vi "Change Bookmarks Type.vi"(8 "Error In":errorcluster, 10 "Data":variant, 11 "State In":T1) -> (0 "Error Out":errorcluster, 3 "State Out":T1)   [LabVIEW 2017, in "Graveyard.lvlib"]
uses:
  Graveyard.lvlib
  State.ctl
  Bookmarks Type.ctl
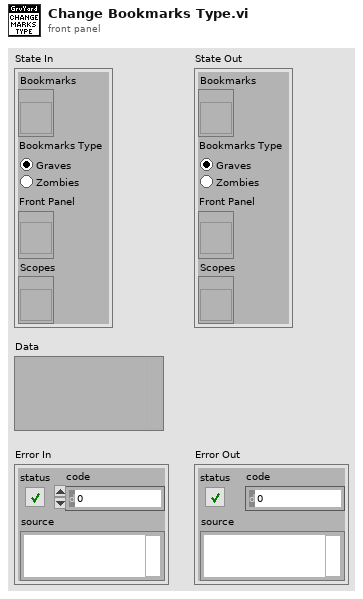
[diagram p1: front panel]
types:
  T1 = typedef "Graveyard.lvlib/State.ctl" = cluster{"Bookmarks":refnum<vi>, "Bookmarks Type":T2, "Front Panel":refnum<vi>, "Scopes":refnum<vi>}
  T2 = typedef "Graveyard.lvlib/Bookmarks Type.ctl" = enum32{"Graves", "Zombies"}
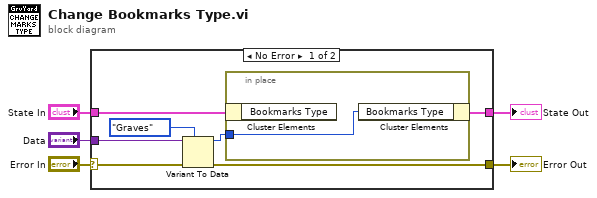
[diagram p0: block diagram]
diagram:
  n1 = case shown="No Error" "Error In" {
    selector: "Error In" -> [w6 w14]
    tunnel: [w10 w15] -> w5
    tunnel: "State In" -> [w9 w15]
    tunnel: "Data" -> [w8 _]
    tunnel: [w7 w14] -> w2
    frame No Error {
      n2 = Variant To Data(error in=w6, type=Bookmarks_Type."Graves" ("Bookmarks Type"), Variant=w8) -> (data=w11:T2, error out=w7:errorcluster)
      n3 = in-place {
        in-place-border: w11 -> [w13]
        n4 = in-place-cluster #1(w9) -> ()  [unwired: 1 out]
        n5 = in-place-cluster #1("Bookmarks Type"=w13) -> (w10:T1)
      }
    }
    frame Error {
    }
  }
  "State Out" <- w5
  "Error Out" <- w2
